vi "CapacitanceEquivalent.vi"(1 "Connect":enum16{"SZEREGOWO", "RÓWNOLEGLE"}(ring) caption="Rodzaj połączenia", 2 "C":dbl[](array[numeric])) -> (0 "C_eq":dbl caption="C_Z  [Farad]" format="%#.2g")   [LabVIEW 2020]
doc: "Ten subVI liczy pojemność zastepczą."
panel:
  # "[Farad]"
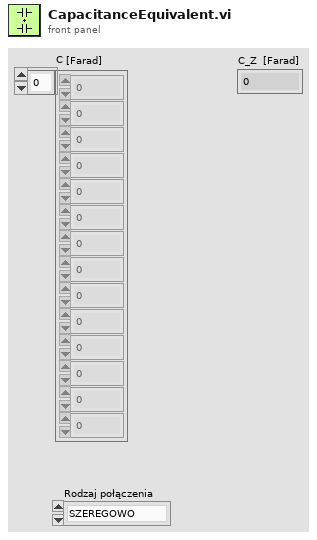
[diagram p1: front panel]
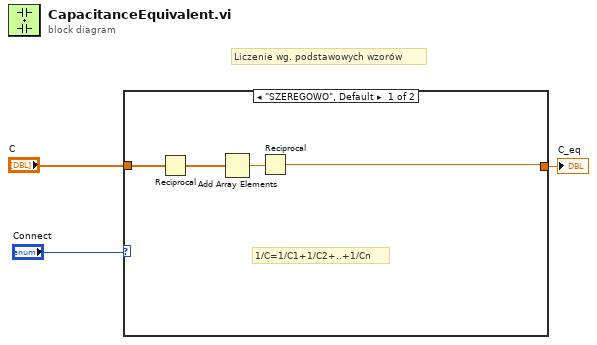
[diagram p0: block diagram]
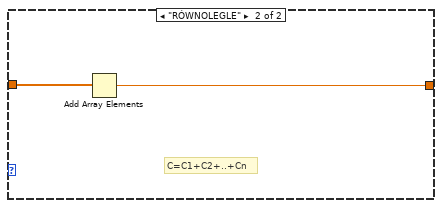
[diagram p2: hidden frame]
diagram:
  # "Liczenie wg. podstawowych wzorów"
  n1 = case shown="\"SZEREGOWO\", Default" "Connect" {
    tunnel: "C" -> [w7 w9]
    tunnel: [w4 w8] -> w1
    frame "SZEREGOWO", Default {
      # "1/C=1/C1+1/C2+..+1/Cn"
      n2 = Reciprocal(x=w7) -> (1/x=w6:dbl[])
      n3 = Add Array Elements(numeric array=w6) -> (sum=w5:dbl)
      n4 = Reciprocal(x=w5) -> (1/x=w4:dbl)
    }
    frame "RÓWNOLEGLE" {
      # "C=C1+C2+..+Cn"
      n5 = Add Array Elements(numeric array=w9) -> (sum=w8:dbl)
    }
  }
  "C_eq" <- w1
